vi "32xx_Decod_OK_WR.vi"(8 "entrée d'erreur":errorcluster caption="Entrée d'erreur", 10 "Entrée Chaîne Caractères":string="0 Local\r", 11 "Visa In":refnum<visa-resource-name>="COM3" caption="Port d'entrée") -> (0 "sortie d'erreur":errorcluster caption="Sortie d'erreur", 2 "Sortie Chaîne Caractères":string="0 OK\r", 3 "Visa Out":refnum<visa-resource-name>="COM3" caption="Port de sortie", 5 "Acknowledge":bool caption="'OK' reçu")   [LabVIEW 2020]
uses:
  <vilib>/Utility/error.llb/Error Cluster From Error Code.vi
  <vilib>/ErrorRing/Error Ring.xnode
panel:
  # "© 2020 elc CORPORATION.  \nALL RIGHTS RESERVED."
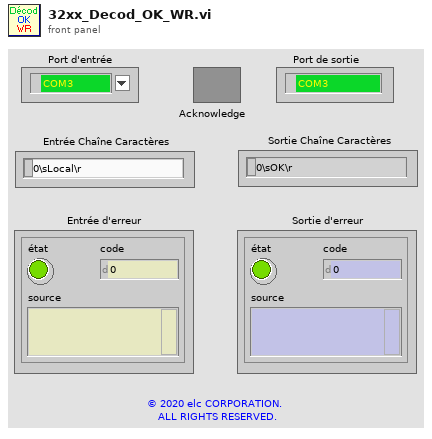
[diagram p1: front panel]
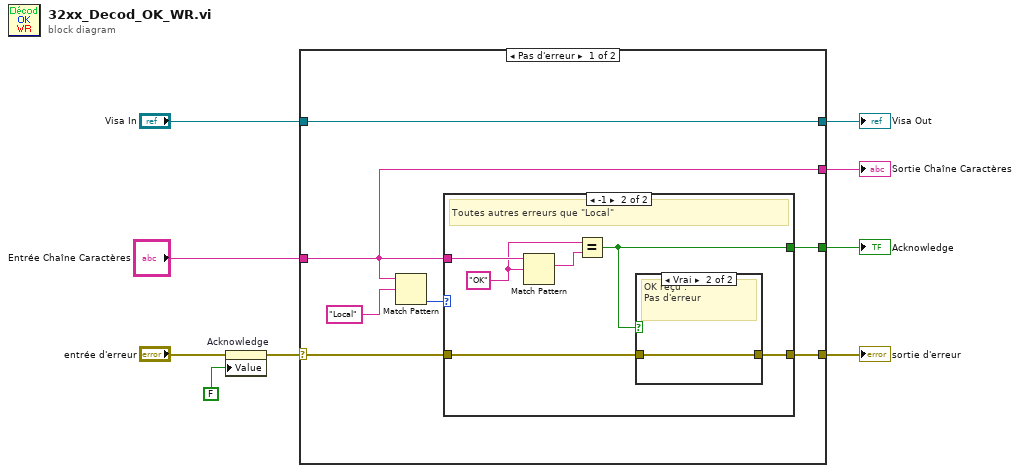
[diagram p0: block diagram]
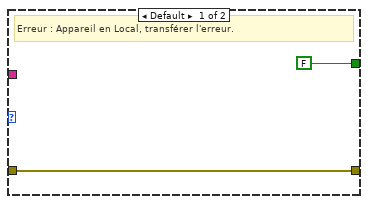
[diagram p2: hidden frame]
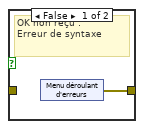
[diagram p3: hidden frame]
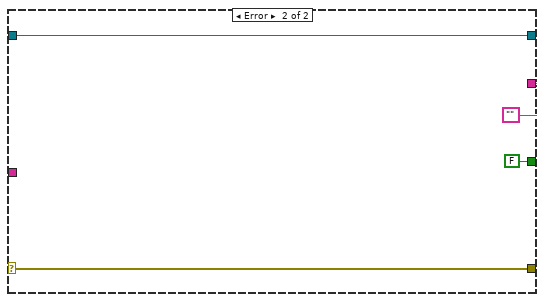
[diagram p4: hidden frame]
diagram:
  n1 = property on="Acknowledge" class="Bool (strict)"(error in="entrée d'erreur", "Value"=FALSE ("'OK' reçu")) -> (error out=w7:errorcluster)  [unwired: 1 in, 1 out]
  n2 = case shown="Pas d'erreur" w7 {
    selector: w7 -> [w13 w33]
    tunnel: [w14 FALSE] -> w5
    tunnel: "Entrée Chaîne Caractères" -> [w12 _]
    tunnel: [w15 w33] -> w2
    tunnel: "Visa In" -> [w16 w32]
    tunnel: [w16 w32] -> w4
    tunnel: [w12 ""] -> w6
    frame No Error {
      n3 = Match Pattern(string=w12, regular expression="Local" ("expression régulière")) -> (offset past match=w10:i32)  [unwired: 1 in, 3 out]
      n4 = case shown="-1" w10 {
        tunnel: [w18 w24] -> w15
        tunnel: [FALSE w23] -> w14
        tunnel: w13 -> [w18 w22]
        tunnel: w12 -> [_ w21]
        frame Default {
          # "Erreur : Appareil en Local, transférer l'erreur."
        }
        frame -1 {
          w19 = "OK" ("expression régulière")
          # "Toutes autres erreurs que \"Local\""
          n5 = Match Pattern(string=w21, regular expression=w19) -> (match substring=w20:string)  [unwired: 1 in, 3 out]
          n6 = Equal?(x=w19, y=w20) -> (x = y?=w23:bool)
          n7 = case shown="Vrai" w23 {
            tunnel: [w25 w30] -> w24
            tunnel: w22 -> [_ w30]
            frame False {
              # "OK non reçu :\nErreur de syntaxe"
              n8 = xnode ("Menu déroulant d'erreurs")() -> ("sortie d'erreur"=w25:errorcluster)
            }
            frame True {
              # "OK reçu :\nPas d'erreur"
            }
          }
        }
      }
    }
    frame Error {
    }
  }
  "sortie d'erreur" <- w2
  "Visa Out" <- w4
  "Acknowledge" <- w5
  "Sortie Chaîne Caractères" <- w6
